vi "GetPersonnel.vi"(7 "LabVIEW Web Service Request":refnum<class "Web Request.lvclass">, 10 "Command":string, 11 "UID":string) -> (2 "Response":string)   [LabVIEW 2015]
uses:
  <vilib>/wsapi/Web Request.lvclass
  TypeDef/PersonnelActions.ctl
panel:
  out "current time":timestamp
  out "postdata":string
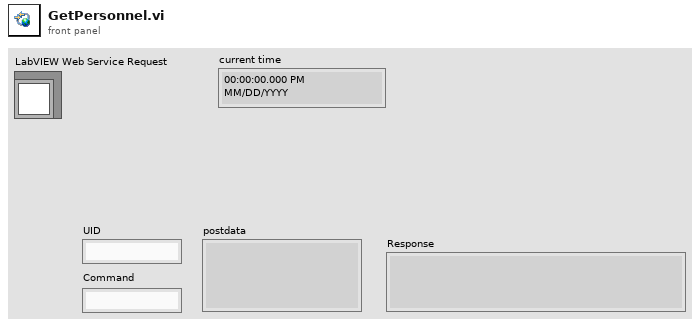
[diagram p1: front panel]
types:
  T1 = typedef "PersonnelActions.ctl" = enum16{"Init", "Read Personnel", "Add Personnel", "Remove Personnel", "Read Name", "Write Name", "Read Role", "Write Role", "Read Requests", "Add Requests", "Remove Requests", "Read PUIDs", "Read PUIDs for Role", "Read All Personnel"}
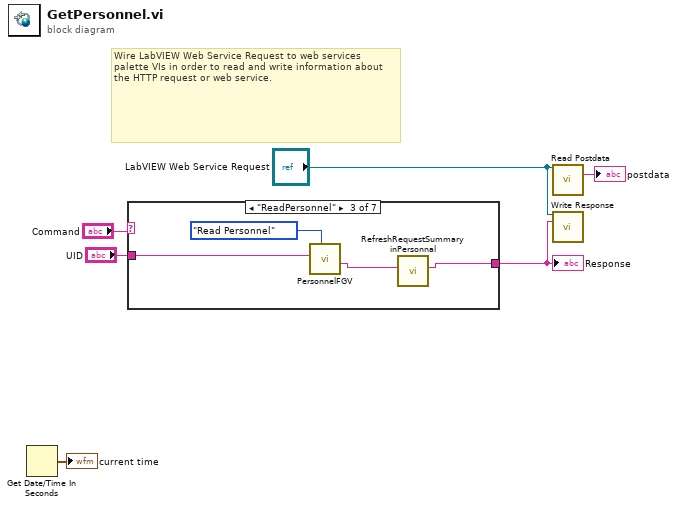
[diagram p0: block diagram]
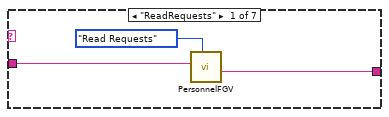
[diagram p2: hidden frame]
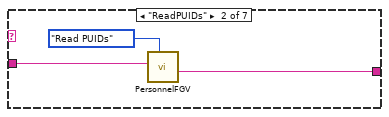
[diagram p3: hidden frame]
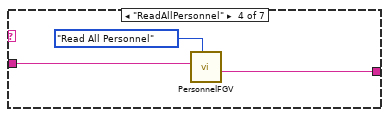
[diagram p4: hidden frame]
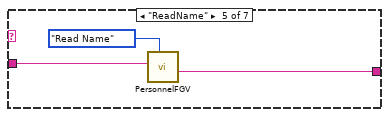
[diagram p5: hidden frame]
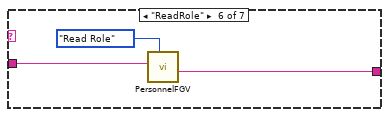
[diagram p6: hidden frame]
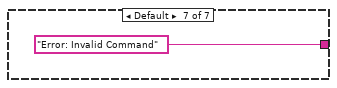
[diagram p7: hidden frame]
diagram:
  # "Wire LabVIEW Web Service Request to web services palette VIs in order to read and write information about the HTTP request or web service."
  n1 = Get Date/Time In Seconds() -> (seconds since 1Jan1904=→"current time":timestamp)
  n2 = case shown="\"ReadPersonnel\"" "Command" {
    tunnel: "UID" -> [w9 w12 w16 w19 w22 w25 _]
    tunnel: [w8 w11 w13 w18 w21 w24 "Error: Invalid Command" ("Data Out")] -> w5
    frame "ReadRequests" {
      n3 = call "PersonnelFGV.vi"("Actions"=PersonnelActions."Read Requests", "PUID"=w9) -> ("Data Out"=w8:string)  [unwired: 8 in, 1 out]
    }
    frame "ReadPUIDs" {
      n4 = call "PersonnelFGV.vi"("Actions"=PersonnelActions."Read PUIDs", "PUID"=w12) -> ("Data Out"=w11:string)  [unwired: 8 in, 1 out]
    }
    frame "ReadPersonnel" {
      n5 = call "PersonnelFGV.vi"("Actions"=PersonnelActions."Read Personnel", "PUID"=w16) -> ("Data Out"=w14:string)  [unwired: 8 in, 1 out]
      n6 = call "RefreshRequestSummaryinPersonnal.vi"("Personnal"=w14) -> ("Personnal"=w13:string)  [unwired: 9 in, 1 out]
    }
    frame "ReadAllPersonnel" {
      n7 = call "PersonnelFGV.vi"("Actions"=PersonnelActions."Read All Personnel", "PUID"=w19) -> ("Data Out"=w18:string)  [unwired: 8 in, 1 out]
    }
    frame "ReadName" {
      n8 = call "PersonnelFGV.vi"("Actions"=PersonnelActions."Read Name", "PUID"=w22) -> ("Data Out"=w21:string)  [unwired: 8 in, 1 out]
    }
    frame "ReadRole" {
      n9 = call "PersonnelFGV.vi"("Actions"=PersonnelActions."Read Role", "PUID"=w25) -> ("Data Out"=w24:string)  [unwired: 8 in, 1 out]
    }
    frame Default {
    }
  }
  "Response" <- w5
  n10 = call <vilib>:"Read Postdata.vi"("LabVIEW Web Service Request"="LabVIEW Web Service Request") -> ("postdata"=→"postdata":string)  [unwired: 12 in, 2 out]
  n11 = call <vilib>:"Write Response.vi"("LabVIEW Web Service Request"="LabVIEW Web Service Request", "response string"=w5) -> ()  [unwired: 12 in, 2 out]
